vi "Test Osciloscope API.vi"() -> ()   [LabVIEW 2020]
doc: "Osciloscope API Tester."
uses:
  TypeDefs/InitializeOsciloscope--cluster.ctl
  TypeDefs/ConfigurateCahnnel--cluster.ctl
  TypeDefs/ReadWaveform--cluster.ctl
  TypeDefs/ReadMeasurementIn--cluster.ctl
  TypeDefs/ReadMeasurementOut--cluster.ctl
  TypeDefs/Read2channelsIn--cluster.ctl
  TypeDefs/Read2ChannlesOut.ctl
  Osciloscope.lvlib
panel:
  out "Read 2 channels Out":T1
  in  "Read 2 channels In":T2={"Channel 1 (1: Channel 1)"=1, "Channel 2 (2: Channel 2)"=2, "Measurement Type (0: Phase)"=0} {"Measurement Type (0: Phase)" items=["Phase", "Delay", "DelayRR", "DelayRF", "DelayFR", "DelayFF"]; "Channel 2 (2: Channel 2)" items=["Channel 1"=1, "Channel 2"=2, "Channel 3"=3, "Channel 4"=4]; "Channel 1 (1: Channel 1)" items=["Channel 1"=1, "Channel 2"=2, "Channel 3"=3, "Channel 4"=4]}
  in  "Read 2 Measurement Channels Osciloscope":bool
  out "Read measurement Out":T3
  in  "Read Measurement In":T4={"Channel (1: Channel 1)"=1, "Measurement Type (0: Frequency)"=0} {"Measurement Type (0: Frequency)" items=["Frequency", "Mean", "Period", "Pulse Duty", "Peak to Peak", "Cycle RMS", "Minimum", "Maximum", "Rise Time", "Fall Time", "Positive Width", "Negative Width", "Amplitude", "Cycle Mean", "High", "Low", "Negative Duty", "Positive Overshoot", "Negative Overshoot", "Cursor Mean", "Burst Width", "Positive Pulse Count", "Negative Pulse Count", "Rising Edge Count", "Falling Edge Count", "Area", "Cycle Area", "RMS", "Cursor RMS"]; "Channel (1: Channel 1)" items=["Channel 1"=1, "Channel 2"=2, "Channel 3"=3, "Channel 4"=4]}
  in  "Read Measurement Osciloscope":bool
  out "Waveform Graph":dbl[](graph)
  in  "ReadWaveform":T5={"Source (0: Channel 1)"=0, "Timeout (10000 ms)"=10000} {"Source (0: Channel 1)" items=["Channel 1", "Channel 2", "Channel 3", "Channel 4", "Math", "Reference A", "Reference B", "Reference C", "Reference D", "FFT"]}
  in  "Read Waveform Osciloscope":bool
  in  "Reset Osciloscope":bool
  in  "Configurate Channel--cluster":T6={"Enable Channel (True)"=TRUE, "Channel (0: Channel 1)"=0, "Vertical Coupling (1: DC)"=1, "Probe Attenuation (10: 10X)"=10, "Vertical Range (10.0 V/div)"=10.0, "Vertical Offset (0.0 divs)"=0.0, "Bandwidth (0: MAX Bandwidth)"=0} {"Bandwidth (0: MAX Bandwidth)" items=["MAX Bandwidth", "Unlimited"]; "Probe Attenuation (10: 10X)" items=["1"=1, "10"=10, "20"=20, "50"=50, "100"=100, "500"=500, "1000"=1000]; "Vertical Coupling (1: DC)" items=["AC", "DC", "Ground"]; "Channel (0: Channel 1)" items=["Channel 1", "Channel 2", "Channel 3", "Channel 4", "Math", "Reference A", "Reference B", "Reference C", "Reference D"]}
  in  "Configure Channel":bool
  in  "Auto Setup Osciloscope":bool
  in  "Close Osciloscope":bool
  in  "Initialize--cluster":T7={"Serial Configuration"={"Baud Rate"=9600, "Parity"=0, "Stop Bits"=10, "Flow Control"=2}, "ID Query? (T: Yes)"=TRUE, "Reset? (T: Yes)"=TRUE} {"Serial Configuration"."Flow Control" items=["None", "XON/XOFF", "RTS/CTS", "XON/XOFF & RTS/CTS", "DTR/DSR", "XON/XOFF & DTR/DSR"]; "Serial Configuration"."Stop Bits" items=["1.0"=10, "1.5"=15, "2.0"=20]; "Serial Configuration"."Parity" items=["None", "Odd", "Even", "Mark", "Space"]; "Serial Configuration"."Baud Rate" items=["300"=300, "600"=600, "1200"=1200, "2400"=2400, "4800"=4800, "9600"=9600, "19200"=19200]}
  in  "Init Osciloscope":bool
  in  "Osciloscopes Avaliables":string(combo)
  in  "Inizializate":bool
  in  "Com Port":refnum<visa-resource-name>
  in  "Set Com Port":bool
  in  "Run as Singleton?":bool
  in  "Show Block Diagram":bool
  in  "Refresh Modules":bool
  out "Active Modules":string[](array[string])
  in  "Stop Module":bool
  in  "Select Module":i32(ring)=-1 caption="Select Module\nTo send Request to" items=["All"=-1]
  in  "Run New Module":bool
  in  "Hide Module Panel":bool
  in  "Show Module Panel":bool
  out "Status":string
  # "This VI tests the API for the Module."
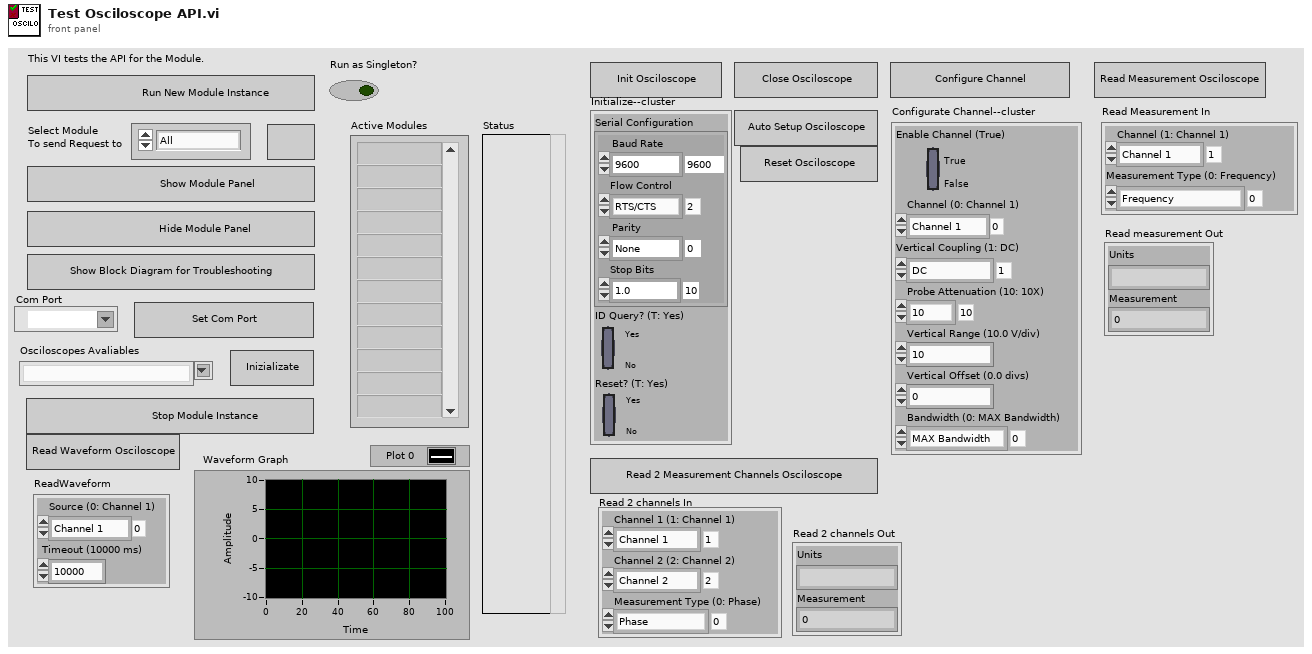
[diagram p1: front panel]
types:
  T1 = typedef "Read2ChannlesOut.ctl" = cluster{"Units":string, "Measurement":dbl}
  T2 = typedef "Read2channelsIn--cluster.ctl" = cluster{"Channel 1 (1: Channel 1)":i32, "Channel 2 (2: Channel 2)":i32, "Measurement Type (0: Phase)":i32}
  T3 = typedef "ReadMeasurementOut--cluster.ctl" = cluster{"Units":string, "Measurement":dbl}
  T4 = typedef "ReadMeasurementIn--cluster.ctl" = cluster{"Channel (1: Channel 1)":i32, "Measurement Type (0: Frequency)":i32}
  T5 = typedef "ReadWaveform--cluster.ctl" = cluster{"Source (0: Channel 1)":u16, "Timeout (10000 ms)":u32}
  T6 = typedef "ConfigurateCahnnel--cluster.ctl" = cluster{"Enable Channel (True)":bool, "Channel (0: Channel 1)":i32, "Vertical Coupling (1: DC)":i32, "Probe Attenuation (10: 10X)":i32, "Vertical Range (10.0 V/div)":dbl, "Vertical Offset (0.0 divs)":dbl, "Bandwidth (0: MAX Bandwidth)":i32}
  T7 = typedef "InitializeOsciloscope--cluster.ctl" = cluster{"Serial Configuration":cluster{"Baud Rate":u32, "Parity":u16, "Stop Bits":u16, "Flow Control":u16}, "ID Query? (T: Yes)":bool, "Reset? (T: Yes)":bool}
  T8 = typedef "Osciloscope.lvlib/Broadcast Events--cluster.ctl" = cluster{"Module Did Init":refnum<user-event>, "Status Updated":refnum<user-event>, "Error Reported":refnum<user-event>, "Module Did Stop":refnum<user-event>, "Update Module Execution Status":refnum<user-event>, "Obtain Osciloscope Name":refnum<user-event>}
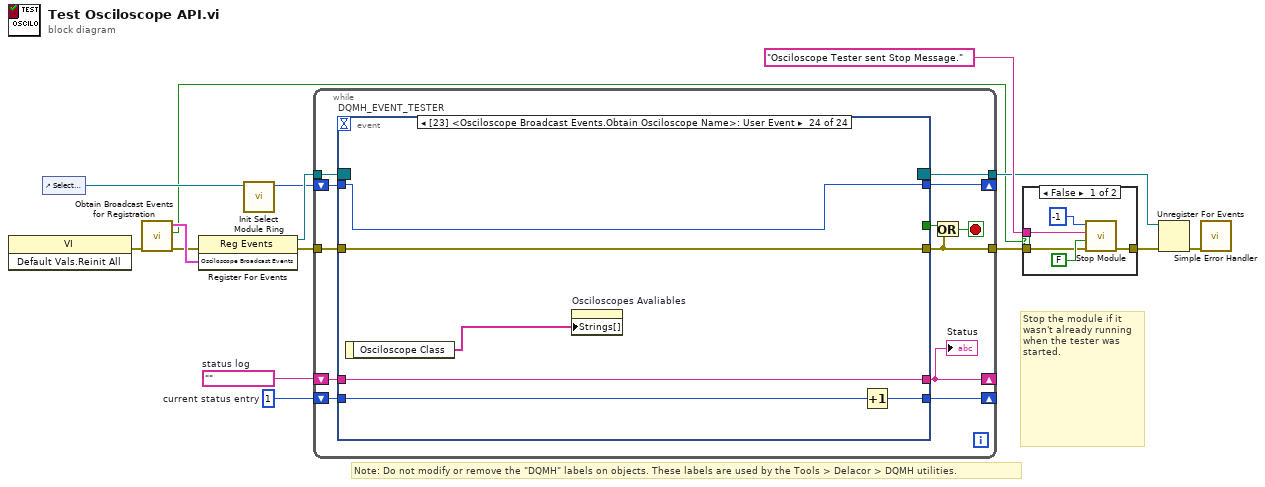
[diagram p0: block diagram]
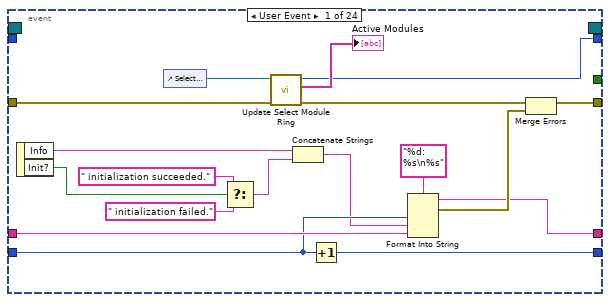
[diagram p3: hidden frame]
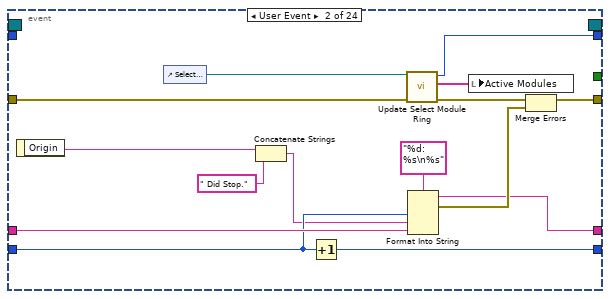
[diagram p4: hidden frame]
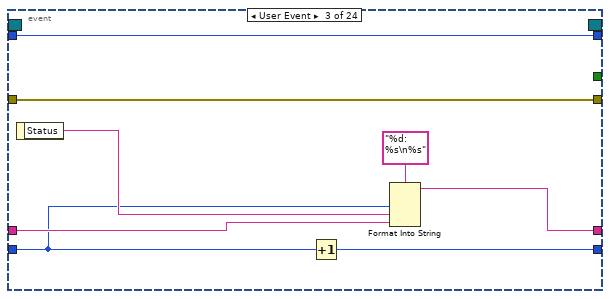
[diagram p5: hidden frame]
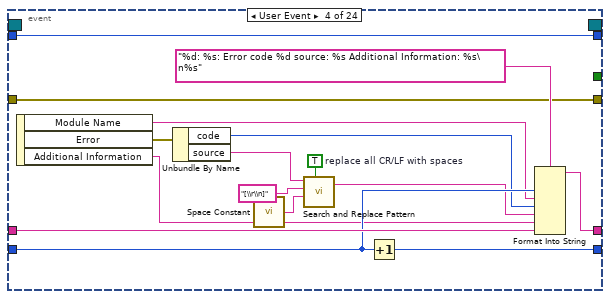
[diagram p6: hidden frame]
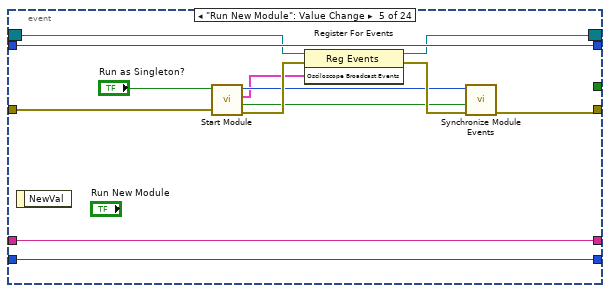
[diagram p7: hidden frame]
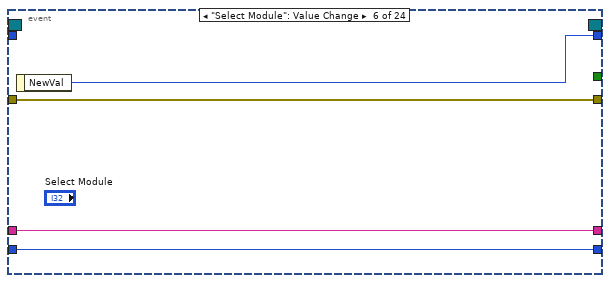
[diagram p8: hidden frame]
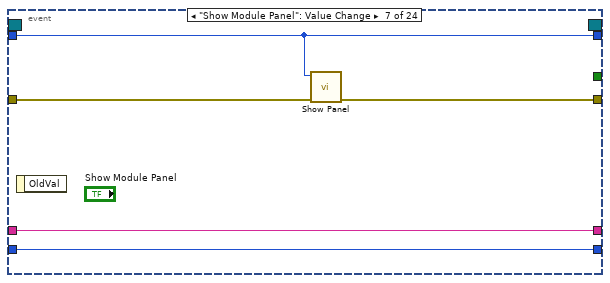
[diagram p9: hidden frame]
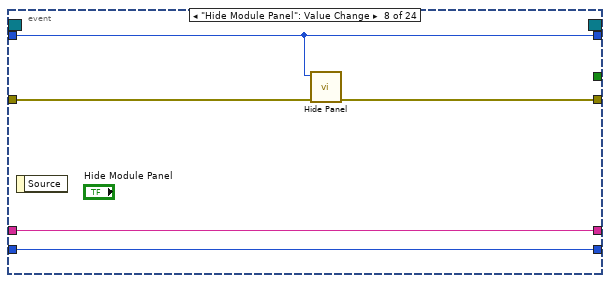
[diagram p10: hidden frame]
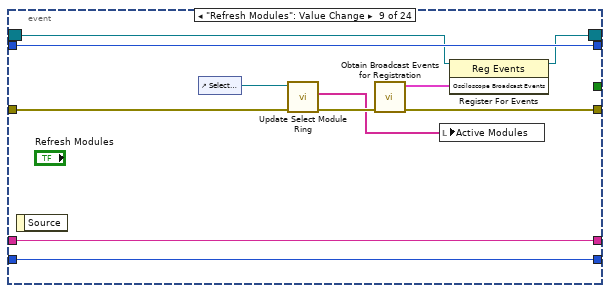
[diagram p11: hidden frame]
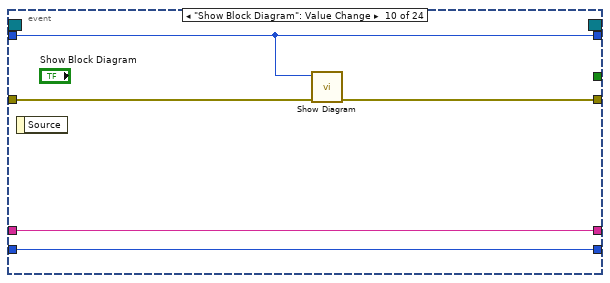
[diagram p12: hidden frame]
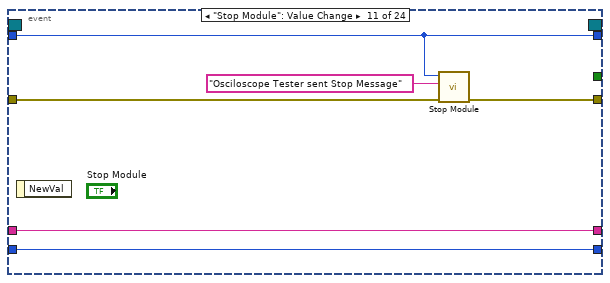
[diagram p13: hidden frame]
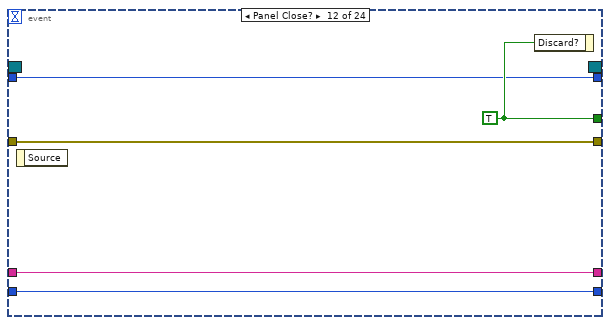
[diagram p14: hidden frame]
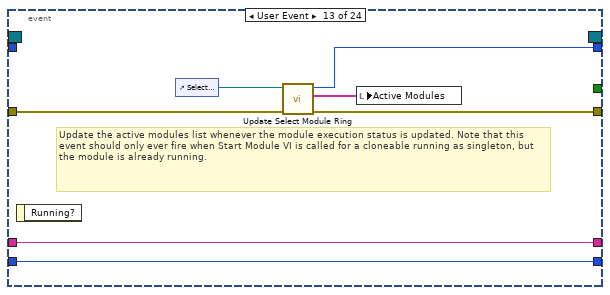
[diagram p15: hidden frame]
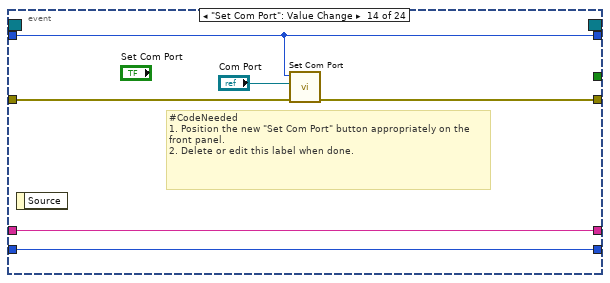
[diagram p16: hidden frame]
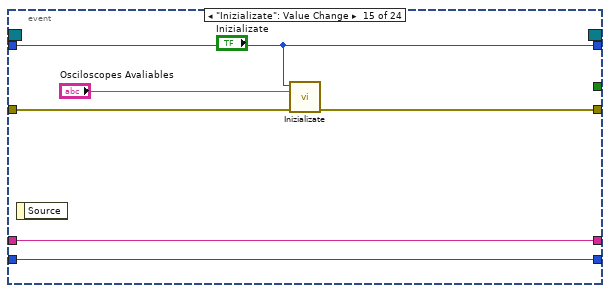
[diagram p17: hidden frame]
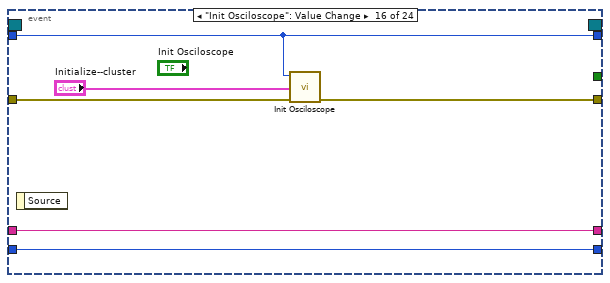
[diagram p18: hidden frame]
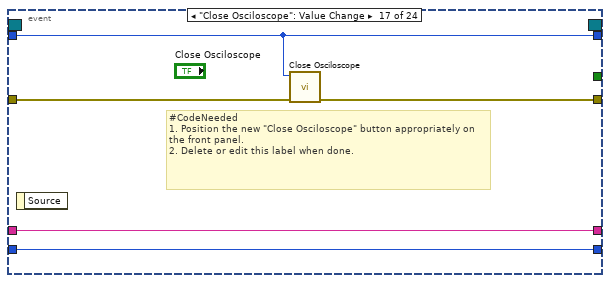
[diagram p19: hidden frame]
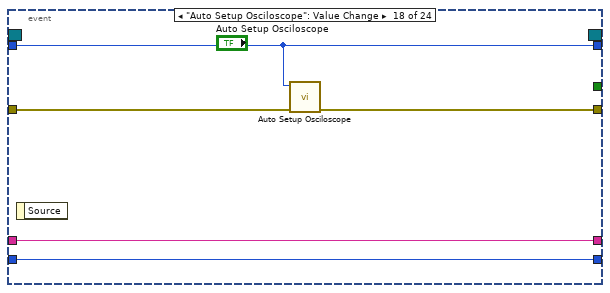
[diagram p20: hidden frame]
diagram:
  w12 = 1  # current status entry
  w13 = ""  # status log
  # "Stop the module if it wasn't already running when the tester was started."
  # "Note: Do not modify or remove the \"DQMH\" labels on objects. These labels are used by the Tools > Delacor > DQMH utilities."
  n1 = invoke class="VI" method="Default Vals.Reinit All"() -> (error out=w5:errorcluster)  [unwired: 3 in, 2 out]
  n2 = control-ref of="Select Module"() -> (w10:refnum<vi>)
  n3 = call "Obtain Broadcast Events for Registration.vi"("error in (no error)"=w5) -> ("error out"=w4:errorcluster, "Already running?"=w3:bool, "Osciloscope Broadcast Events"=w9:T8)  [unwired: 8 in]
  n4 = register-events(error in=w4, w9) -> (reference out=w15:refnum<event-registration>, error out=w8:errorcluster)  [unwired: 1 in]
  n5 = call "Init Select Module Ring.vi"("Select Module Ring Ref"=w10) -> ("Value for All Modules"=w11:i32)  [unwired: 8 in, 2 out]
  n6 = while {
    tunnel: w15 -> [w27]
    tunnel: [w16] -> w2
    tunnel: w8 -> [w25]
    shift-right: [w21] -> _
    shift-left: w13 -> [w23]
    shift-right: [w22] -> _
    shift-left: w12 -> [w24]
    shift-right: [w18] -> _
    shift-left: w11 -> [w19]
    tunnel: [w17] -> w6
    stop <- w20 stop-if-true
    n7 = event "DQMH_EVENT_TESTER" shown="[23] <Osciloscope Broadcast Events.Obtain Osciloscope Name>: User Event" {
      selector: w27 -> [_ _ _ _ w91 _ _ _ w117 _ _ _ _ _ _ _ _ _ _ _ _ _ _ _]
      dyn-events: [_ _ _ _ w90 _ _ _ w116 _ _ _ _ _ _ _ _ _ _ _ _ _ _ _] -> w17
      timeout: _ -> [_ _ _ _ _ _ _ _ _ _ _ _ _ _ _ _ _ _ _ _ _ _ _ _]
      tunnel: [_ _ _ _ _ _ _ _ _ _ _ w138 _ _ _ _ _ _ _ _ _ _ _ _] -> w26
      tunnel: [w35 w52 w68 w74 w89 w101 w105 w110 w113 w124 w129 w137 w141 w148 w154 w160 w165 w170 w176 w181 w188 w195 w202 w211] -> w16
      tunnel: w25 -> [w37 w54 w68 w74 w92 w101 w106 w111 w118 w127 w130 w137 w142 w151 w157 w163 w168 w173 w179 w184 w191 w198 w205 w211]
      tunnel: w24 -> [w42 w57 w61 w80 w94 w99 w103 w108 w121 w125 w132 w135 w144 w149 w155 w161 w166 w171 w177 w182 w189 w196 w203 w209]
      tunnel: w23 -> [w43 w58 w64 w82 w95 w100 w104 w109 w122 w126 w133 w136 w145 w150 w156 w162 w167 w172 w178 w183 w190 w197 w204 w207]
      tunnel: [w40 w55 w65 w77 w95 w100 w104 w109 w122 w126 w133 w136 w145 w150 w156 w162 w167 w172 w178 w183 w190 w197 w204 w207] -> w21
      tunnel: [w41 w56 w67 w83 w94 w99 w103 w108 w121 w125 w132 w135 w144 w149 w155 w161 w166 w171 w177 w182 w189 w196 w203 w208] -> w22
      tunnel: w19 -> [_ _ w62 w84 w93 _ w102 w107 w120 w123 w131 w134 _ w147 w153 w159 w164 w169 w175 w180 w187 w194 w201 w210]
      tunnel: [w32 w49 w62 w84 w93 w98 w102 w107 w120 w123 w131 w134 w140 w147 w153 w159 w164 w169 w175 w180 w187 w194 w201 w210] -> w18
      event User Event {
        n8 = event-data() -> ("Info"=w39:string, "Init?"=w29:bool)  [unwired: 1 in]
        n9 = control-ref of="Select Module"() -> (w34:refnum<vi>)
        n10 = Select(t=" initialization succeeded.", s=w29, f=" initialization failed.") -> (s? t:f=w28:string)
        n11 = call "Update Select Module Ring.vi"("error in (no error)"=w37, "Select Module Ring Ref"=w34) -> ("error out"=w36:errorcluster, "Active Modules (Array)"=→"Active Modules":string[], "New Module Ring Value"=w32:i32)  [unwired: 7 in]
        n12 = Concatenate Strings(w39, w28) -> (w38:string)
        n13 = Increment(x=w42) -> (x+1=w41:i32)
        n14 = Format Into String(format string="%d: %s\n%s", w42, w38, w43) -> (resulting string=w40:string, error out=w45:errorcluster)  [unwired: 2 in]
        n15 = Merge Errors(w36, w45) -> (w35:errorcluster)
      }
      event User Event {
        n16 = event-data() -> ("Origin"=w47:string)  [unwired: 1 in]
        n17 = control-ref of="Select Module"() -> (w51:refnum<vi>)
        n18 = Concatenate Strings(w47, " Did Stop.") -> (w46:string)
        n19 = Increment(x=w57) -> (x+1=w56:i32)
        n20 = call "Update Select Module Ring.vi"("error in (no error)"=w54, "Select Module Ring Ref"=w51) -> ("error out"=w53:errorcluster, "Active Modules (Array)"=w50:string[], "New Module Ring Value"=w49:i32)  [unwired: 7 in]
        n21 = Format Into String(format string="%d: %s\n%s", w57, w46, w58) -> (resulting string=w55:string, error out=w60:errorcluster)  [unwired: 2 in]
        n22 = local write "Active Modules"(w50) -> ()
        n23 = Merge Errors(w53, w60) -> (w52:errorcluster)
      }
      event User Event {
        n24 = event-data() -> ("Status"=w63:string)  [unwired: 1 in]
        n25 = Increment(x=w61) -> (x+1=w67:i32)
        n26 = Format Into String(format string="%d: %s\n%s", w61, w63, w64) -> (resulting string=w65:string)  [unwired: 2 in, 1 out]
      }
      event User Event {
        w78 = TRUE  # replace all CR/LF with spaces
        n27 = event-data() -> ("Module Name"=w72:string, "Error"=w71:errorcluster, "Additional Information"=w69:string)  [unwired: 1 in]
        n28 = Unbundle By Name(w71) -> ("code"=w73:i32, "source"=w75:string)
        n29 = call <vilib>:"Space Constant.vi"() -> ("String"=w79:string)
        n30 = call <vilib>:"Search and Replace Pattern.vi"("string"=w75, "regular expression (\"\")"="[\\r\\n]" ("regular expression (\"\")"), "replace string (\"\")"=w79, "replace all? (F)"=w78) -> ("result string"=w76:string)  [unwired: 1 in, 1 out]
        n31 = Increment(x=w80) -> (x+1=w83:i32)
        n32 = Format Into String(format string="%d: %s: Error code %d source: %s Additional Information: %s\n%s", w80, w72, w73, w76, w69, w82) -> (resulting string=w77:string)  [unwired: 2 in, 1 out]
      }
      event "Run New Module": Value Change {
        n33 = event-data() -> ()  [unwired: 1 in, 1 out]
        n34 = call "Start Module.vi"("error in"=w92, "Run as Singleton? (F)"="Run as Singleton?") -> ("error out"=w96:errorcluster, "Wait for Event Sync?"=w87:bool, "Osciloscope Broadcast Events"=w86:T8, "Module ID"=w88:i32)  [unwired: 6 in]
        n35 = register-events(reference=w91, error in=w96, w86) -> (reference out=w90:refnum<event-registration>, error out=w97:errorcluster)
        n36 = call "Synchronize Module Events.vi"("error in"=w97, "Wait for Event Sync?"=w87, "Module ID in"=w88) -> ("error out"=w89:errorcluster)  [unwired: 7 in, 1 out]
      }
      event "Select Module": Value Change {
        n37 = event-data() -> ("NewVal"=w98:i32)  [unwired: 1 in]
      }
      event "Show Module Panel": Value Change {
        n38 = event-data() -> ()  [unwired: 1 in, 1 out]
        n39 = call "Show Panel.vi"("error in (no error)"=w106, "Module ID"=w102) -> ("error out"=w105:errorcluster)  [unwired: 9 in]
      }
      event "Hide Module Panel": Value Change {
        n40 = event-data() -> ()  [unwired: 1 in, 1 out]
        n41 = call "Hide Panel.vi"("error in (no error)"=w111, "Module ID"=w107) -> ("error out"=w110:errorcluster)  [unwired: 9 in]
      }
      event "Refresh Modules": Value Change {
        n42 = event-data() -> ()  [unwired: 1 in, 1 out]
        n43 = control-ref of="Select Module"() -> (w119:refnum<vi>)
        n44 = call "Update Select Module Ring.vi"("error in (no error)"=w118, "Select Module Ring Ref"=w119) -> ("error out"=w114:errorcluster, "Active Modules (Array)"=w112:string[])  [unwired: 7 in, 1 out]
        n45 = call "Obtain Broadcast Events for Registration.vi"("error in (no error)"=w114) -> ("error out"=w113:errorcluster, "Osciloscope Broadcast Events"=w115:T8)  [unwired: 8 in, 1 out]
        n46 = local write "Active Modules"(w112) -> ()
        n47 = register-events(reference=w117, w115) -> (reference out=w116:refnum<event-registration>)  [unwired: 1 in, 1 out]
      }
      event "Show Block Diagram": Value Change {
        n48 = event-data() -> ()  [unwired: 1 in, 1 out]
        n49 = call "Show Diagram.vi"("error in (no error)"=w127, "Module ID"=w123) -> ("error out"=w124:errorcluster)  [unwired: 9 in]
      }
      event "Stop Module": Value Change {
        n50 = event-data() -> ()  [unwired: 1 in, 1 out]
        n51 = call "Stop Module.vi"("error in (no error)"=w130, "Origin"="Osciloscope Tester sent Stop Message", "Module ID"=w131) -> ("error out"=w129:errorcluster)  [unwired: 8 in]
      }
      event Panel Close? {
        w138 = TRUE ("Discard?")
        n52 = event-data() -> ()  [unwired: 1 in, 1 out]
        n53 = event-data("Discard?"=w138) -> ()  [unwired: 1 in, 1 out]
      }
      event User Event {
        # "Update the active modules list whenever the module execution status is updated. Note that this event should only ever fire when Start Module VI is called for a cloneable running as singleton, but the module is already running."
        n54 = event-data() -> ()  [unwired: 1 in, 1 out]
        n55 = control-ref of="Select Module"() -> (w143:refnum<vi>)
        n56 = call "Update Select Module Ring.vi"("error in (no error)"=w142, "Select Module Ring Ref"=w143) -> ("error out"=w141:errorcluster, "Active Modules (Array)"=w139:string[], "New Module Ring Value"=w140:i32)  [unwired: 7 in]
        n57 = local write "Active Modules"(w139) -> ()
      }
      event "Set Com Port": Value Change {
        # "#CodeNeeded\n1. Position the new \"Set Com Port\" button appropriately on the front panel.\n2. Delete or edit this label when done."
        n58 = event-data() -> ()  [unwired: 1 in, 1 out]
        n59 = call "Set Com Port.vi"("error in"=w151, "Com Port"="Com Port", "Module ID"=w147) -> ("error out"=w148:errorcluster)  [unwired: 8 in]
      }
      event "Inizializate": Value Change {
        n60 = event-data() -> ()  [unwired: 1 in, 1 out]
        n61 = call "Inizializate.vi"("error in"=w157, "Osciloscope"="Osciloscopes Avaliables", "Module ID"=w153) -> ("error out"=w154:errorcluster)  [unwired: 8 in]
      }
      event "Init Osciloscope": Value Change {
        n62 = event-data() -> ()  [unwired: 1 in, 1 out]
        n63 = call "Init Osciloscope.vi"("error in"=w163, "Initialize--cluster"="Initialize--cluster", "Module ID"=w159) -> ("error out"=w160:errorcluster)  [unwired: 8 in]
      }
      event "Close Osciloscope": Value Change {
        # "#CodeNeeded\n1. Position the new \"Close Osciloscope\" button appropriately on the front panel.\n2. Delete or edit this label when done."
        n64 = event-data() -> ()  [unwired: 1 in, 1 out]
        n65 = call "Close Osciloscope.vi"("error in"=w168, "Module ID"=w164) -> ("error out"=w165:errorcluster)  [unwired: 9 in]
      }
      event "Auto Setup Osciloscope": Value Change {
        n66 = event-data() -> ()  [unwired: 1 in, 1 out]
        n67 = call "Auto Setup Osciloscope.vi"("error in"=w173, "Module ID"=w169) -> ("error out"=w170:errorcluster)  [unwired: 9 in]
      }
      event "Configure Channel": Value Change {
        # "#CodeNeeded\n1. Position the new \"Configure Channel\" button appropriately on the front panel.\n2. Delete or edit this label when done."
        n68 = event-data() -> ()  [unwired: 1 in, 1 out]
        n69 = call "Configure Channel.vi"("error in"=w179, "Configurate Channel--cluster"="Configurate Channel--cluster", "Module ID"=w175) -> ("error out"=w176:errorcluster)  [unwired: 8 in]
      }
      event "Reset Osciloscope": Value Change {
        # "#CodeNeeded\n1. Position the new \"Reset Osciloscope\" button appropriately on the front panel.\n2. Delete or edit this label when done."
        n70 = event-data() -> ()  [unwired: 1 in, 1 out]
        n71 = call "Reset Osciloscope.vi"("error in"=w184, "Module ID"=w180) -> ("error out"=w181:errorcluster)  [unwired: 9 in]
      }
      event "Read Waveform Osciloscope": Value Change {
        # "#CodeNeeded\n1. Position the new \"Read Waveform Osciloscope\" button appropriately on the front panel.\n2. Delete or edit this label when done."
        n72 = event-data() -> ()  [unwired: 1 in, 1 out]
        n73 = call "Read Waveform Osciloscope.vi"("error in"=w191, "ReadWaveform"="ReadWaveform", "Module ID"=w187) -> ("error out"=w188:errorcluster, "Waveform Graph"=→"Waveform Graph":dbl[])  [unwired: 6 in, 1 out]
      }
      event "Read Measurement Osciloscope": Value Change {
        n74 = event-data() -> ()  [unwired: 1 in, 1 out]
        n75 = call "Read Measurement Osciloscope.vi"("error in"=w198, "Read Measurement In"="Read Measurement In", "Module ID"=w194) -> ("error out"=w195:errorcluster, "Read measurement Out"=→"Read measurement Out":T3)  [unwired: 6 in, 1 out]
      }
      event "Read 2 Measurement Channels Osciloscope": Value Change {
        # "#CodeNeeded\n1. Position the new \"Read 2 Measurement Channels Osciloscope\" button appropriately on the front panel.\n2. Delete or edit this label when done."
        n76 = event-data() -> ()  [unwired: 1 in, 1 out]
        n77 = call "Read 2 Measurement Channels Osciloscope.vi"("error in"=w205, "Read 2 channels In"="Read 2 channels In", "Module ID"=w201) -> ("error out"=w202:errorcluster, "Read 2 channels Out"=→"Read 2 channels Out":T1)  [unwired: 6 in, 1 out]
      }
      event User Event {
        n78 = event-data() -> ("Osciloscope Class"=w206:string[])  [unwired: 1 in]
        n79 = property on="Osciloscopes Avaliables" class="CmbBox"("Strings[]"=w206) -> ()  [unwired: 2 in, 2 out]
        n80 = Increment(x=w209) -> (x+1=w208:i32)
      }
    }
    "Status" <- w21
    n81 = Or(x=w26, y=w16) -> (x .or. y?=w20:bool)
  }
  n82 = case shown="False" w3 {
    tunnel: [w216 w217] -> w14
    tunnel: "Osciloscope Tester sent Stop Message." ("Origin") -> [w215 _]
    tunnel: w2 -> [w212 w217]
    frame False {
      n83 = call "Stop Module.vi"("error in (no error)"=w212, "Wait for Module to stop? (F)"=FALSE ("Wait for Module to stop?"), "Origin"=w215, "Module ID"=-1 ("Stop all")) -> ("error out"=w216:errorcluster)  [unwired: 7 in]
    }
    frame True {
    }
  }
  n84 = Unregister For Events(event registration refnum=w6, error in=w14) -> (error out=w1:errorcluster)
  n85 = call <vilib>:"Simple Error Handler.vi"("error in (no error)"=w1) -> ()  [unwired: 4 in, 5 out]
